vi "Test Listen 2.vi"() -> ()   [LabVIEW 2014, in "Arduino SoftwareSerial Wrapper.lvlib"]
uses:
  Arduino SoftwareSerial Wrapper.lvlib
panel:
  out "Is Listening? 2":bool
  out "Is Listening?":bool
  out "Error Out":errorcluster
  in  "Error In":errorcluster
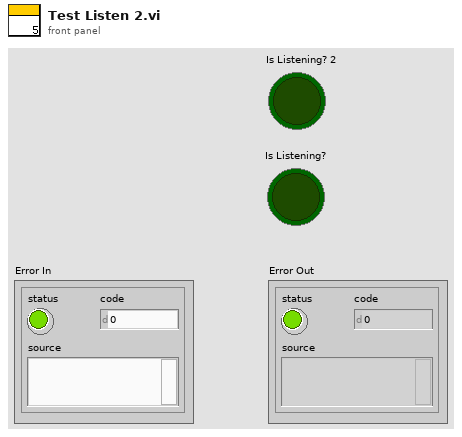
[diagram p1: front panel]
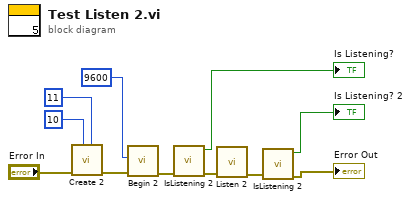
[diagram p0: block diagram]
diagram:
  n1 = call "Create 2.vi"("arduino RX pin"=u8 11 ("arduino TX pin"), "arduino TX pin"=u8 10 ("arduino RX pin"), "Error In"="Error In") -> ("Error Out"=w8:errorcluster)  [unwired: 8 in]
  n2 = call "Begin 2.vi"("Error In"=w8, "Baudrate"=u16 9600) -> ("Error Out"=w6:errorcluster)  [unwired: 8 in]
  n3 = call "IsListening 2.vi"("Error In"=w6) -> ("Error Out"=w5:errorcluster, "Is Listening?"=→"Is Listening?":bool)  [unwired: 9 in]
  n4 = call "Listen 2.vi"("Error In"=w5) -> ("Error Out"=w4:errorcluster)  [unwired: 10 in]
  n5 = call "IsListening 2.vi"("Error In"=w4) -> ("Error Out"=→"Error Out":errorcluster, "Is Listening?"=→"Is Listening? 2":bool)  [unwired: 9 in]
